vi "InitializeOCUCommunication.vi"(2 "error in (no error)":errorcluster, 3 "Boat Type":T1(ring)) -> (0 "error out":errorcluster, 1 "NetworkStreamReader out":refnum<class "NetworkStreamReader.lvclass">)   [LabVIEW 2013]
doc: "Initializes stream for communication with the OCU\n\nAuthored: Victoria Coleman 03/28/14"
uses:
  RIO-OCU_Comm/NetworkStreams/Reader/NetworkStreamReader.lvclass
  RIO-OCU_Comm/ToRIO.ctl
  OCU/CommandMessages.ctl
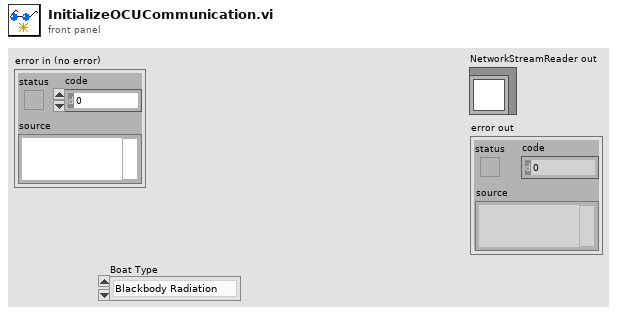
[diagram p1: front panel]
types:
  T1 = enum16{"Blackbody Radiation", "Little boats", "Simulation", "Damn Yankee"}
  T2 = typedef "ToRIO.ctl" = cluster{"Commands":T3, "Variant":variant}
  T3 = typedef "CommandMessages.ctl" = enum16{"Pass", "OverrideMode", "Add mission", "Delete mission", "Change constants"}
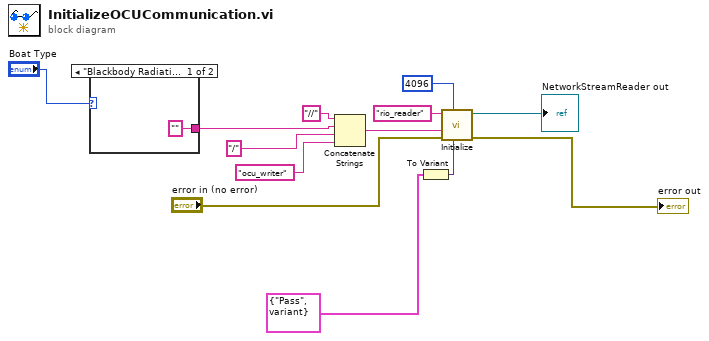
[diagram p0: block diagram]
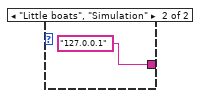
[diagram p2: hidden frame]
diagram:
  n1 = case shown="\"Blackbody Radiation\", Default" "Boat Type" {
    tunnel: ["" "127.0.0.1"] -> w1
    frame "Blackbody Radiation", Default {
    }
    frame "Little boats", "Simulation" {
    }
  }
  n2 = Concatenate Strings("//" ("string"), w1, "/", "ocu_writer" ("string")) -> (w9:string)
  n3 = To Variant(anything=T2 {"Commands"=enum."Pass", "Variant"=variant} ("To RIO")) -> (Variant=w12:variant)
  n4 = call "Initialize.vi"("Default return"=w12, "reader buffer size"=4096 ("writer buffer size"), "error in (no error)"="error in (no error)", "writer url"=w9, "reader name"="rio_reader" ("writer name")) -> ("error out"=→"error out":errorcluster, "NetworkStreamReader out"=→"NetworkStreamReader out":refnum<class "NetworkStreamReader.lvclass">)  [unwired: 5 in]
